vi "Read Log File Path.vi"(8 "error in (no error)":errorcluster, 11 "Abstract Log Init Parameters in":refnum<class "Abstract Log Init Parameters.lvclass">) -> (0 "error out":errorcluster, 2 "Log File Path":path, 3 "Abstract Log Init Parameters out":refnum<class "Abstract Log Init Parameters.lvclass">)   [LabVIEW 2020, in "Abstract Log Init Parameters.lvclass"]
uses:
  Abstract Log Init Parameters.lvclass
  Abstract Log Init Parameters.lvclass/Abstract Log Init Parameters.ctl
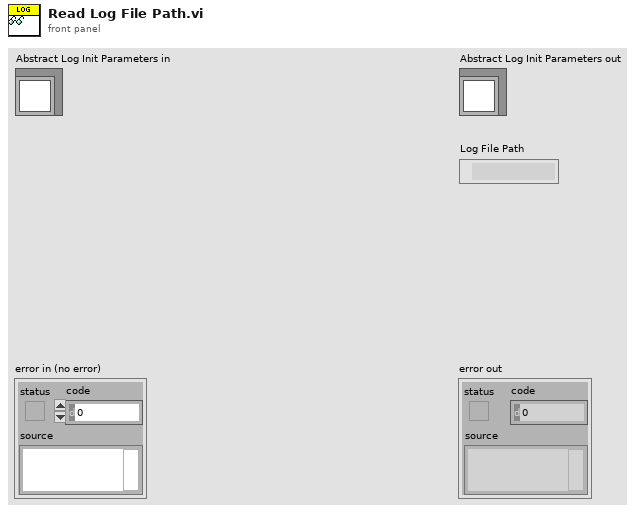
[diagram p1: front panel]
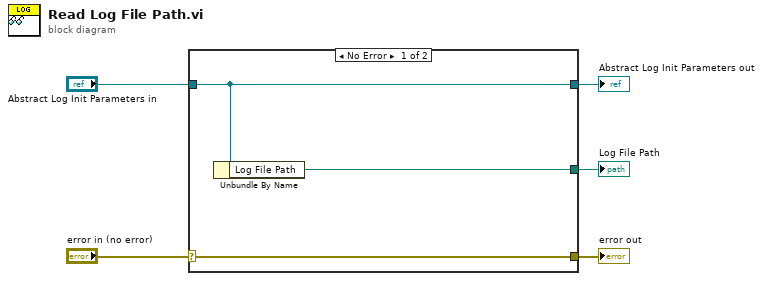
[diagram p0: block diagram]
diagram:
  n1 = case shown="No Error" "error in (no error)" {
    selector: "error in (no error)" -> [w8 w9]
    tunnel: [w8 w9] -> w4
    tunnel: [w7 w10] -> w2
    tunnel: "Abstract Log Init Parameters in" -> [w7 w10]
    tunnel: [w6 _] -> w1
    frame No Error {
      n2 = Unbundle By Name(w7) -> ("Log File Path"=w6:path)
    }
    frame Error {
    }
  }
  "error out" <- w4
  "Abstract Log Init Parameters out" <- w2
  "Log File Path" <- w1
